vi "SaveToML.vi"(0 "X1":i32[](array[numeric]), 1 "Y1":i32[](array[numeric]), 3 "X2":i32[](array[numeric]), 4 "Y2":i32[](array[numeric]), 6 "X3":i32[](array[numeric]), 7 "Y3":i32[](array[numeric]), 8 "band touch":u32(colorbox), 9 "path":path, 10 "ball touch":u32(colorbox), 11 "W":i16, 12 "line":string, 13 "H":i16, 15 "MATLAB Script":string) -> (23 "Analyse":string)   [LabVIEW 2019]
doc: "Ce VI génère le string “Analyse” contenant le script MATLAB qui doit être exécuté.\n\nIl prend en entrée : \n- Les entiers “W” et “H” correspondant à la largeur et la hauteur des images (en pixels);\n- Le chemin du dossier contenant la séquence d’images;\n- “ball touch” : la valeur en hexadécimal de la couleur d’affichage de l’impact la boule du joueur et une autre boule sur MATLAB. Cette couleur est choisie par l’utilisateur dans l’interface Labview.\n- “band touch” : la valeur en hexadécimal de la couleur d’affichage de l’impact entre la boule du joueur et la bande du billard sur MATLAB. Cette couleur est choisie par l’utilisateur dans l’interface Labview.\n- Le string “line” accessible depuis l’interface Labview par l’utilisateur. Dans ce string, l’utilisateur indique le type de ligne choisi pour afficher les trajectoires des boules sur MATLAB.\n- Les coordonnées des boules rouge (X1,Y1), jaune (X2,Y2), blanche (X3,Y3) sur chaque image. Les coordonnées sont sous forme de 6 tableaux, dont la taille est le nombre d’images de la séquence.\n- Le string “MATLAB Script” qui contient notre code MATLAB.\n\nIl renvoie en sortie un string “Analyse” contenant le script destiné à être envoyé à MATLAB. Le string Analyse rassemble toutes les entrées du VI dans un long string respectant l’écriture MATLAB."
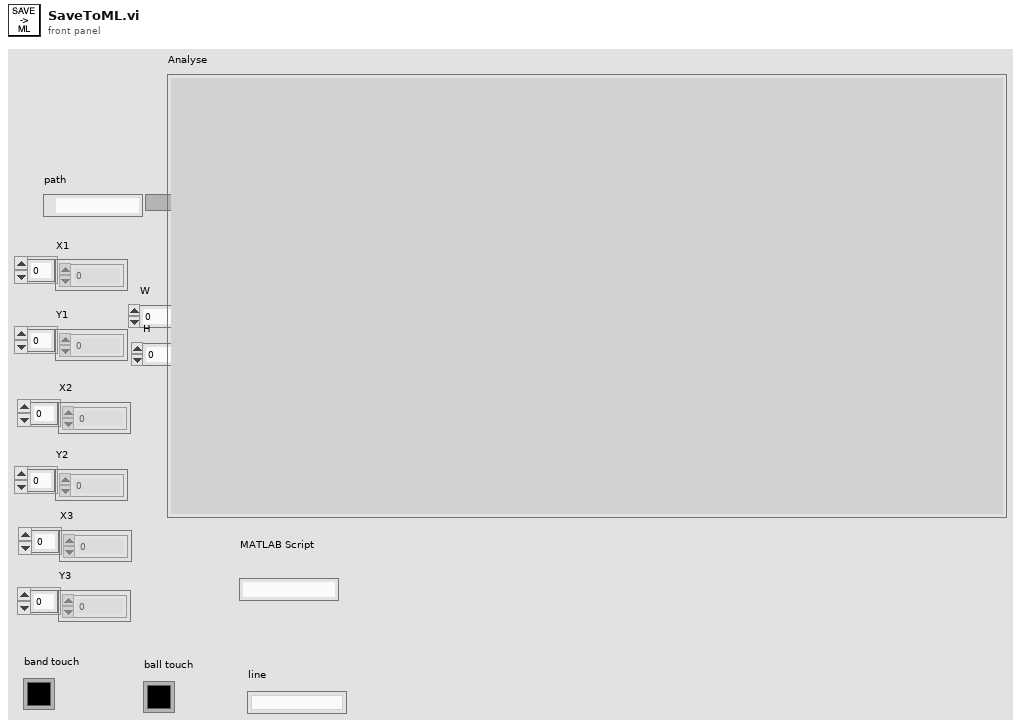
[diagram p1: front panel]
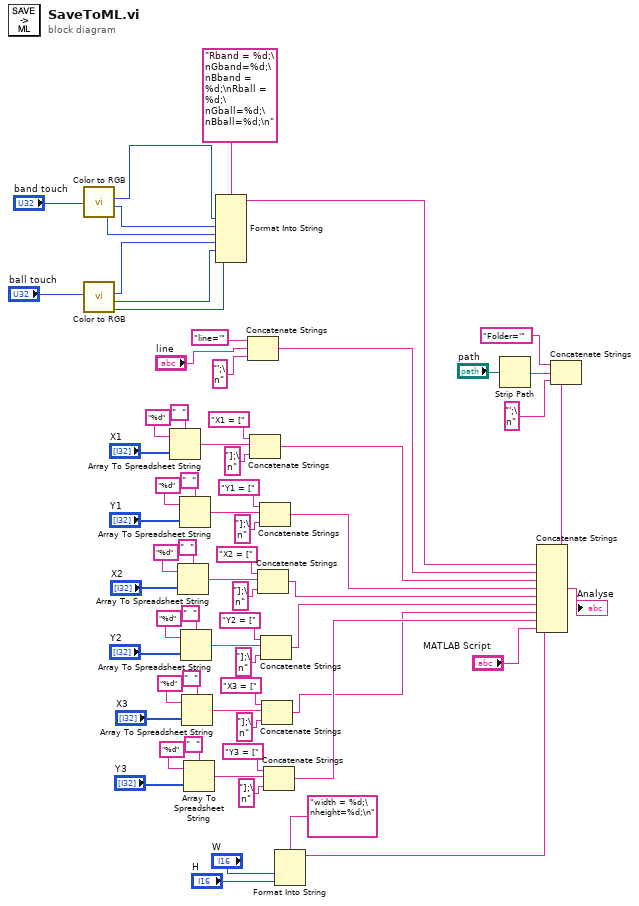
[diagram p0: block diagram]
diagram:
  n1 = call <vilib>:"Color to RGB.vi"("Color"="band touch") -> ("R"=w12:u8, "G"=w11:u8, "B"=w10:u8)  [unwired: 1 out]
  n2 = call <vilib>:"Color to RGB.vi"("Color"="ball touch") -> ("R"=w8:u8, "G"=w7:u8, "B"=w6:u8)  [unwired: 1 out]
  n3 = Array To Spreadsheet String(delimiter (Tab)="  ", array="X1", 3:"%d" ("format string")) -> (spreadsheet string=w29:string)
  n4 = Array To Spreadsheet String(delimiter (Tab)="  ", array="X2", 3:"%d" ("format string")) -> (spreadsheet string=w39:string)
  n5 = Array To Spreadsheet String(delimiter (Tab)="  ", array="Y1", 3:"%d" ("format string")) -> (spreadsheet string=w34:string)
  n6 = Array To Spreadsheet String(delimiter (Tab)="  ", array="Y2", 3:"%d" ("format string")) -> (spreadsheet string=w44:string)
  n7 = Array To Spreadsheet String(delimiter (Tab)="  ", array="X3", 3:"%d" ("format string")) -> (spreadsheet string=w49:string)
  n8 = Array To Spreadsheet String(delimiter (Tab)="  ", array="Y3", 3:"%d" ("format string")) -> (spreadsheet string=w54:string)
  n9 = Format Into String(format string="Rband = %d;\nGband=%d;\nBband = %d;\nRball = %d;\nGball=%d;\nBball=%d;\n", w12, w11, w10, w8, w7, w6) -> (resulting string=w4:string)  [unwired: 2 in, 1 out]
  n10 = Concatenate Strings("line='" ("string"), "line", "';\n" ("string")) -> (w14:string)
  n11 = Concatenate Strings("X1 = [" ("string"), w29, "];\n" ("string")) -> (w62:string)
  n12 = Concatenate Strings("X2 = [" ("string"), w39, "];\n" ("string")) -> (w64:string)
  n13 = Concatenate Strings("Y1 = [" ("string"), w34, "];\n" ("string")) -> (w63:string)
  n14 = Concatenate Strings("Y2 = [" ("string"), w44, "];\n" ("string")) -> (w65:string)
  n15 = Concatenate Strings("X3 = [" ("string"), w49, "];\n" ("string")) -> (w66:string)
  n16 = Concatenate Strings("Y3 = [" ("string"), w54, "];\n" ("string")) -> (w67:string)
  n17 = Format Into String(format string="width = %d;\nheight=%d;\n", "W", "H") -> (resulting string=w2:string)  [unwired: 2 in, 1 out]
  n18 = Strip Path(path="path") -> (name=w18:string)  [unwired: 1 out]
  n19 = Concatenate Strings("Folder='", w18, "';\n") -> (w5:string)
  n20 = Concatenate Strings(w2, w5, w4, w14, w62, w63, w64, w65, w66, w67, "MATLAB Script") -> (→"Analyse":string)
